vi "LINE_2.vi"() -> ()   [LabVIEW 2019]
panel:
  in  "LINE_2_in":string
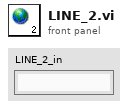
[diagram p1: front panel]
diagram:
